vi "Configure Jitter Spectrum.vi"(0 "VISA resource name":refnum<visa-resource-name>, 1 "Jitter Spectrum Vertical Span (8%)":dbl=8.0, 2 "Jitter Spectrum Vertical Unit (0: VRMS)":i32(ring) items=["VRMS", "Decibel"], 5 "Jitter Spectrum Horizontal Center (50E+3 Hz)":dbl=50000.0, 7 "Jitter Spectrum Horizontal Span (100E+3 Hz)":dbl=100000.0, 9 "Jitter Spectrum Vertical Center (0%)":dbl, 11 "error in (no error)":errorcluster, 12 "Jitter Spectrum Window Transform (0: Hanning)":i32(ring) items=["Hanning", "Flattop", "Rectangular", "Blackman-Harris"]) -> (4 "VISA resource name out":refnum<visa-resource-name>, 15 "error out":errorcluster)   [LabVIEW 2015, in "Agilent 2000 3000 X-Series.lvlib"]
doc: "Configures the Jitter Spectrum feature. Use the <b>Configure Jitter Analysis</b> VI to enable this feature.\n\n<b>Note:</b>\nThis VI is specific to the 6000-X Series oscilloscopes. These features are not available on other models."
uses:
  <instrlib>/Agilent 2000 3000 X-Series/Agilent 2000 3000 X-Series.lvlib
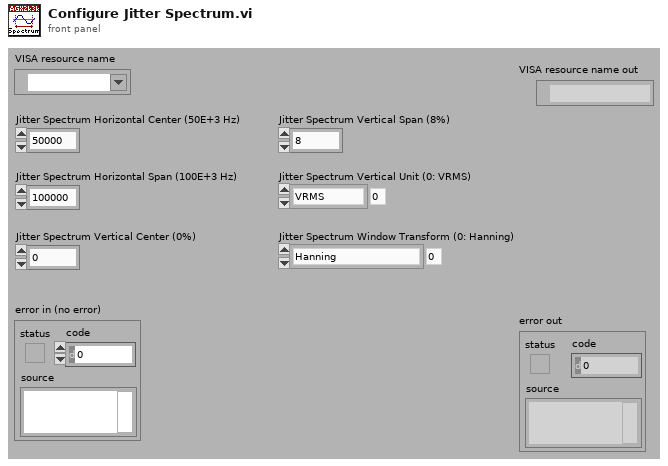
[diagram p1: front panel]
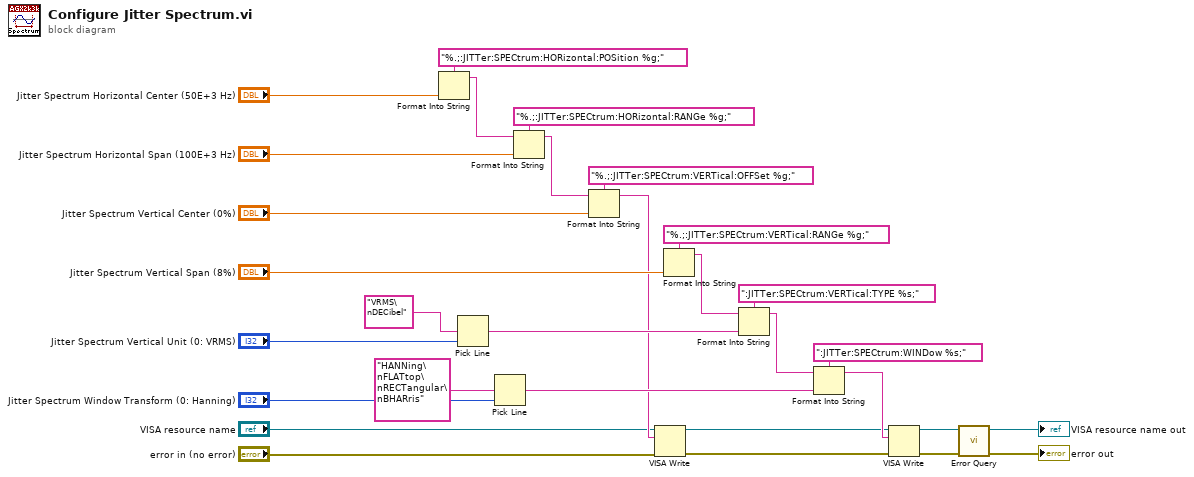
[diagram p0: block diagram]
diagram:
  n1 = Format Into String(format string="%.;:JITTer:SPECtrum:HORizontal:POSition %g;", "Jitter Spectrum Horizontal Center (50E+3 Hz)") -> (resulting string=w12:string)  [unwired: 2 in, 1 out]
  n2 = Pick Line(multi-line string="VRMS\nDECibel", line index="Jitter Spectrum Vertical Unit (0: VRMS)") -> (output string=w17:string)  [unwired: 1 in]
  n3 = Pick Line(multi-line string="HANNing\nFLATtop\nRECTangular\nBHARris", line index="Jitter Spectrum Window Transform (0: Hanning)") -> (output string=w15:string)  [unwired: 1 in]
  n4 = Format Into String(format string="%.;:JITTer:SPECtrum:HORizontal:RANGe %g;", initial string=w12, "Jitter Spectrum Horizontal Span (100E+3 Hz)") -> (resulting string=w11:string)  [unwired: 1 in, 1 out]
  n5 = Format Into String(format string="%.;:JITTer:SPECtrum:VERTical:OFFSet %g;", initial string=w11, "Jitter Spectrum Vertical Center (0%)") -> (resulting string=w13:string)  [unwired: 1 in, 1 out]
  n6 = VISA Write(VISA resource name="VISA resource name", write buffer=w13, error in (no error)="error in (no error)") -> (VISA resource name out=w6:refnum<visa-resource-name>, error out=w5:errorcluster)  [unwired: 1 out]
  n7 = Format Into String(format string="%.;:JITTer:SPECtrum:VERTical:RANGe %g;", "Jitter Spectrum Vertical Span (8%)") -> (resulting string=w10:string)  [unwired: 2 in, 1 out]
  n8 = Format Into String(format string=":JITTer:SPECtrum:VERTical:TYPE %s;", initial string=w10, w17) -> (resulting string=w9:string)  [unwired: 1 in, 1 out]
  n9 = Format Into String(format string=":JITTer:SPECtrum:WINDow %s;", initial string=w9, w15) -> (resulting string=w20:string)  [unwired: 1 in, 1 out]
  n10 = VISA Write(VISA resource name=w6, write buffer=w20, error in (no error)=w5) -> (VISA resource name out=w4:refnum<visa-resource-name>, error out=w3:errorcluster)  [unwired: 1 out]
  n11 = call <instrlib>:"Error Query.vi"("error in (no error)"=w3, "VISA resource name"=w4) -> ("error out"=→"error out":errorcluster, "VISA resource name out"=→"VISA resource name out":refnum<visa-resource-name>)  [unwired: 6 in, 2 out]
